vi "Generate Final Report.vi"(8 "error in":errorcluster) -> (0 "error out":errorcluster)   [LabVIEW 2018, in "Report Generation.lvlib"]
uses:
  Report Generation.lvlib
  <vilib>/Utility/NIReport.llb/Report Type.ctl
  <vilib>/Utility/file.llb/Read Delimited Spreadsheet (string).vi
  <vilib>/addons/_office/excel.llb/Excel Easy Table (str).vi
  <vilib>/Utility/NIReport.llb/NI_report.lvclass
  <vilib>/Utility/NIReport.llb/NI_ReportGenerationCore.lvlib
  <vilib>/addons/_office/NI_ReportGenerationToolkit.lvlib
  <vilib>/Utility/NIReport.llb/Excel/NI_Excel.lvclass
panel:
  out "all rows 2":string[][](array[string])
  out "all rows":string[][][](array[string])
  out "filenames":string[](array[string])
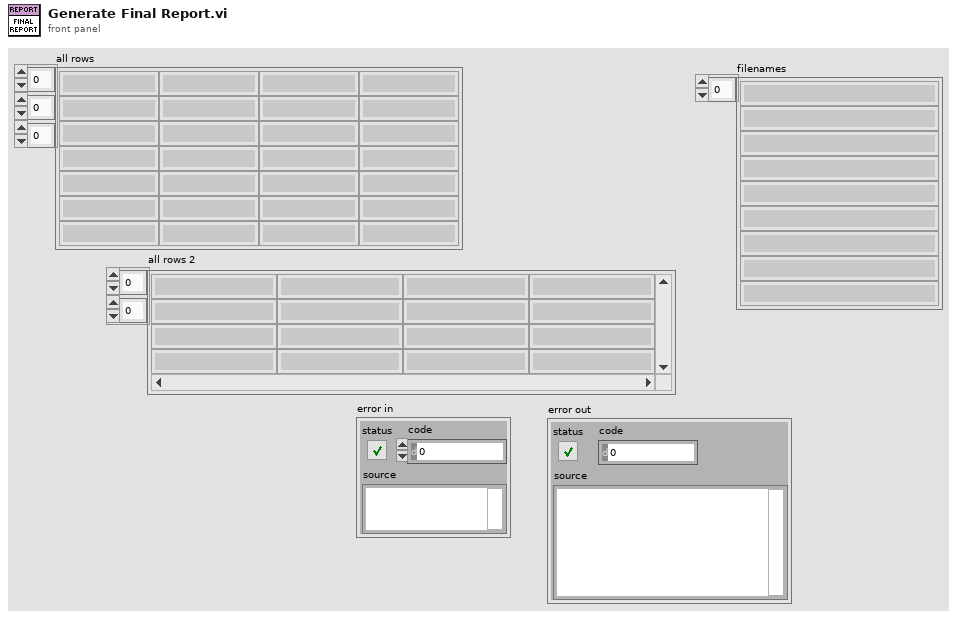
[diagram p1: front panel]
types:
  T1 = enum16{"open", "replace", "create", "open or create", "replace or create", "replace or create with confirmation"}
  T2 = typedef "NI_ReportGenerationCore.lvlib/Report Type.ctl" = enum16{"HTML", "Word", "Excel"}
  T3 = enum16{"maximized", "minimized", "normal", "no change"}
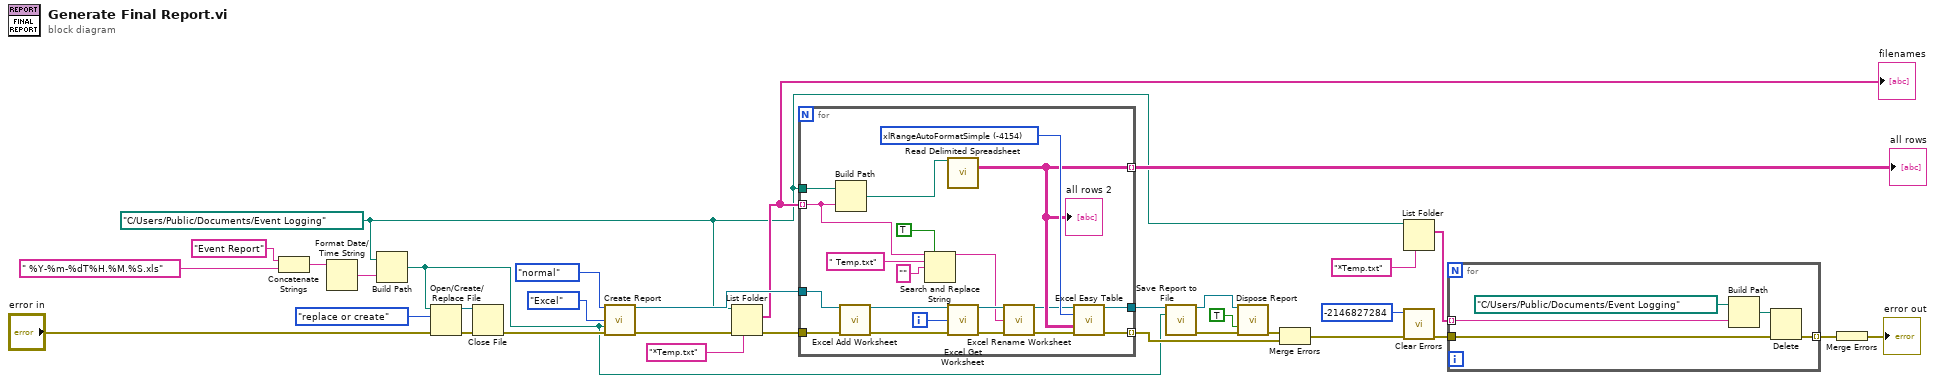
[diagram p0: block diagram]
diagram:
  w5 = path "C:/Users/Public/Documents/Event Logging" ("Path")
  n1 = Concatenate Strings("Event Report" ("title"), " %Y-%m-%dT%H.%M.%S.xls" ("time format string (%c)")) -> (w11:string)
  n2 = Format Date/Time String(time format string (%c)=w11) -> (date/time string=w13:string)  [unwired: 2 in]
  n3 = Build Path(base path=w5, name or relative path=w13) -> (appended path=w9:path)
  n4 = Open/Create/Replace File(file path (use dialog)=w9, error in="error in", operation (0:open)=T1."replace or create") -> (refnum out=w17:refnum<file>, error out=w18:errorcluster)  [unwired: 3 in, 1 out]
  n5 = Close File(refnum=w17, error in=w18) -> (error out=w16:errorcluster)  [unwired: 1 out]
  n6 = call <vilib>:"Create Report.vi"("window state (normal)"=T3."normal", "report type"=Report_Type."Excel", "template (empty)"=w9, "error in (no error)"=w16) -> ("report out"=w30:refnum<class "NI_report.lvclass">, "error out"=w29:errorcluster)  [unwired: 10 in]
  n7 = List Folder(path=w5, pattern="*Temp.txt", error in=w29) -> (filenames=w14:string[], error out=w28:errorcluster)  [unwired: 1 in, 2 out]
  "filenames" <- w14
  n8 = for {
    tunnel: w14 -> [w33] mode=indexing
    tunnel: w5 -> [w52]
    tunnel: [w45] -> w26 mode=indexing
    tunnel: w30 -> [w47]
    tunnel: w28 -> [w46]
    tunnel: [w51] -> w27 mode=indexing
    tunnel: [w49] -> w25
    i -> [w42]
    w50 = -4154 items=["xlRangeAutoFormat3DEffects1"=13, "xlRangeAutoFormat3DEffects2"=14, "xlRangeAutoFormatAccounting1"=4, "xlRangeAutoFormatAccounting2"=5, "xlRangeAutoFormatAccounting3"=6, "xlRangeAutoFormatAccounting4"=17, "xlRangeAutoFormatClassic1"=1, "xlRangeAutoFormatClassic2"=2, "xlRangeAutoFormatClassic3"=3, "xlRangeAutoFormatColor1"=7, "xlRangeAutoFormatColor2"=8, "xlRangeAutoFormatColor3"=9, "xlRangeAutoFormatList1"=10, "xlRangeAutoFormatList2"=11, "xlRangeAutoFormatList3"=12, "xlRangeAutoFormatLocalFormat1"=15, "xlRangeAutoFormatLocalFormat2"=16, "xlRangeAutoFormatLocalFormat3"=19, "xlRangeAutoFormatLocalFormat4"=20, "xlRangeAutoFormatReport1"=21, "xlRangeAutoFormatReport2"=22, "xlRangeAutoFormatReport3"=23, "xlRangeAutoFormatReport4"=24, "xlRangeAutoFormatReport5"=25, "xlRangeAutoFormatReport6"=26, "xlRangeAutoFormatReport7"=27, "xlRangeAutoFormatReport8"=28, "xlRangeAutoFormatReport9"=29, "xlRangeAutoFormatReport10"=30, "xlRangeAutoFormatClassicPivotTable"=31, "xlRangeAutoFormatTable1"=32, "xlRangeAutoFormatTable2"=33, "xlRangeAutoFormatTable3"=34, "xlRangeAutoFormatTable4"=35, "xlRangeAutoFormatTable5"=36, "xlRangeAutoFormatTable6"=37, "xlRangeAutoFormatTable7"=38, "xlRangeAutoFormatTable8"=39, "xlRangeAutoFormatTable9"=40, "xlRangeAutoFormatTable10"=41, "xlRangeAutoFormatPTNone"=42, "xlRangeAutoFormatNone"=-4142, "xlRangeAutoFormatSimple"=-4154] ("auto format (none)")
    n9 = Build Path(base path=w52, name or relative path=w33) -> (appended path=w48:path)
    n10 = call <vilib>:"Excel Add Worksheet.vi"("report in"=w47, "error in (no error)"=w46) -> ("report out"=w44:refnum<class "NI_report.lvclass">, "error out"=w43:errorcluster)  [unwired: 12 in]
    n11 = Search and Replace String(replace all?=TRUE ("replace all? (F)"), input string=w33, search string=" Temp.txt" ("pattern"), replace string="" ("replace string (\"\")")) -> (result string=w36:string)  [unwired: 4 in, 3 out]
    n12 = call-poly <vilib>:"Read Delimited Spreadsheet.vi"("file path (dialog if empty)"=w48) -> ("all rows"=w45:string[][])  [unwired: 9 in, 5 out]
    "all rows 2" <- w45
    n13 = call <vilib>:"Excel Get Worksheet.vi"("report in"=w44, "worksheet index (0)"=w42, "error in (no error)"=w43) -> ("report out"=w41:refnum<class "NI_report.lvclass">, "error out"=w40:errorcluster)  [unwired: 11 in]
    n14 = call <vilib>:"Excel Rename Worksheet.vi"("report in"=w41, "worksheet name (\"\")"=w36, "error in (no error)"=w40) -> ("report out"=w39:refnum<class "NI_report.lvclass">, "error out"=w38:errorcluster)  [unwired: 11 in]
    n15 = call-poly <vilib>:"Excel Easy Table.vi"("report in"=w39, "auto format (none)"=w50, "text data"=w45, "error in (no error)"=w38) -> ("report out"=w49:refnum<class "NI_report.lvclass">, "error out"=w51:errorcluster)  [unwired: 7 in, 3 out]
  }
  "all rows" <- w26
  n16 = call-dynamic "Save Report to File.vi"("report in"=w25, "report file path"=w9) -> ("report out"=w22:refnum<class "NI_report.lvclass">, "error out"=w20:errorcluster)  [unwired: 12 in]
  n17 = call-dynamic "Dispose Report.vi"("report in"=w22, "save changes? (F)"=TRUE, "error in (no error)"=w20) -> ("error out"=w19:errorcluster)  [unwired: 12 in]
  n18 = Merge Errors(w19, w27) -> (w2:errorcluster)
  n19 = List Folder(path=w5, pattern="*Temp.txt") -> (filenames=w4:string[])  [unwired: 2 in, 3 out]
  n20 = call <vilib>:"Clear Errors.vi"("error in (no error)"=w2, "specific error code to clear (0: all)"=-2146827284) -> ("error out"=w1:errorcluster)  [unwired: 4 in, 1 out]
  n21 = for {
    tunnel: [w54] -> w8 mode=indexing
    tunnel: w1 -> [w55]
    tunnel: w4 -> [w53] mode=indexing
    n22 = Build Path(base path=path "C:/Users/Public/Documents/Event Logging" ("path"), name or relative path=w53) -> (appended path=w56:path)
    n23 = Delete(path (use dialog)=w56, error in=w55) -> (error out=w54:errorcluster)  [unwired: 3 in, 2 out]
  }
  n24 = Merge Errors(w8) -> (→"error out":errorcluster)
